vi "Fetch Measurement (Residual FM).vi"(8 "error in (no error)":errorcluster, 11 "VISA resource name":refnum<visa-resource-name>) -> (0 "error out":errorcluster, 2 "Residual FM (Hz)":dbl, 3 "VISA resource name out":refnum<visa-resource-name>)   [LabVIEW 2014, in "Agilent ESA PSA Series.lvlib"]
doc: "Returns the results of the last measurement (Residual FM) and does not initiate data acquisition.\n\n<B>Note:</B>\n\nThis VI is only valid for the Log Plot functionality of the Phase noise personality."
uses:
  Agilent ESA PSA Series.lvlib
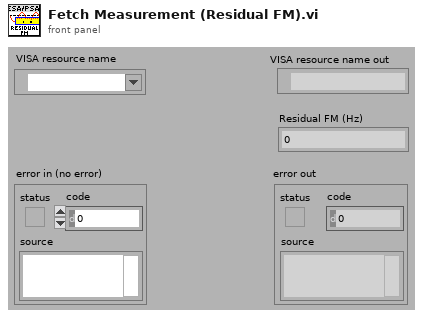
[diagram p1: front panel]
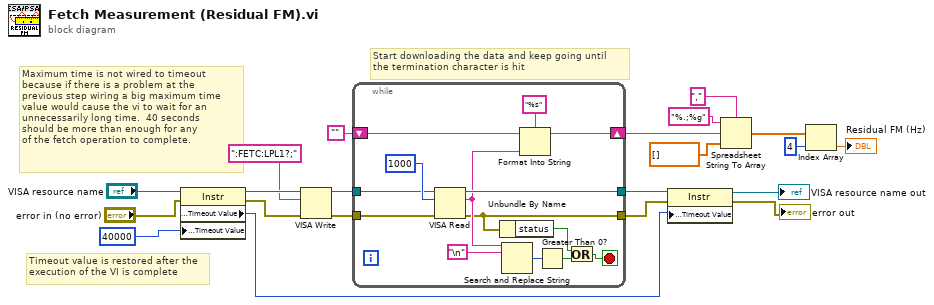
[diagram p0: block diagram]
diagram:
  # "Maximum time is not wired to timeout\nbecause if there is a problem at the\nprevious step wiring a big maximum time\nvalue would cause the vi to wait for an\nunnecessarily long time.  40 seconds\nshould be more than enough for any\nof the fetch operation to complete."
  # "Timeout value is restored after the\nexecution of the VI is complete"
  # "Start downloading the data and keep going until\nthe termination character is hit"
  n1 = property on="Property Node" class="Instr"(reference="VISA resource name", error in="error in (no error)", "General Settings:Timeout Value"=u32 40000) -> (reference out=w18:refnum<visa-resource-name>, error out=w19:errorcluster, "General Settings:Timeout Value"=w15:u32)
  n2 = VISA Write(VISA resource name=w18, write buffer=":FETC:LPL1?;" ("string (\"\")"), error in (no error)=w19) -> (VISA resource name out=w9:refnum<visa-resource-name>, error out=w8:errorcluster)  [unwired: 1 out]
  n3 = while {
    tunnel: [w34] -> w17
    tunnel: [w22] -> w16
    tunnel: w9 -> [w33]
    tunnel: w8 -> [w32]
    shift-right: [w28] -> w6
    shift-left: "" -> [w27]
    stop <- w24 stop-if-true
    n4 = VISA Read(VISA resource name=w33, byte count=u32 1000, error in (no error)=w32) -> (VISA resource name out=w34:refnum<visa-resource-name>, read buffer=w29:string, error out=w22:errorcluster)  [unwired: 1 out]
    n5 = Unbundle By Name(w22) -> ("status"=w25:bool)
    n6 = Search and Replace String(input string=w29, search string="\n") -> (number of replacements=w30:i32)  [unwired: 6 in, 3 out]
    n7 = Format Into String(format string="%s", initial string=w27, w29) -> (resulting string=w28:string)  [unwired: 1 in, 1 out]
    n8 = Greater Than 0?(x=w30) -> (x > 0?=w23:bool)
    n9 = Or(x=w25, y=w23) -> (x .or. y?=w24:bool)
  }
  n10 = property on="Property Node" class="Instr"(reference=w17, error in=w16, "General Settings:Timeout Value"=w15) -> (reference out=→"VISA resource name out":refnum<visa-resource-name>, error out=→"error out":errorcluster)
  n11 = Spreadsheet String To Array(delimiter (Tab)=",", format string="%.;%g", spreadsheet string=w6, array type (2D Dbl)=dbl[] []) -> (array=w3:dbl[])
  n12 = Index Array(array=w3, index=4) -> (element=→"Residual FM (Hz)":dbl)
